vi "Actor Core.vi"(8 "error in":errorcluster, 11 "Dispatcher in":refnum<class "Dispatcher.lvclass">) -> (0 "error out":errorcluster, 3 "Actor out":refnum<class "Actor.lvclass">)   [LabVIEW 2013, in "Dispatcher.lvclass"]
doc: "(<B>Filename</B>: Actor Framework.lvlib:Actor.lvclass:Actor Core.vi)\n\nReceives messages to the actor, reacts to them, and initiates any error handling that may shut the actor down.\n\nDescendant classes may override this VI to append parallel tasks for the actor to complete while it handles messages. Overrides use the Call Parent Method node."
uses:
  Dispatcher.lvclass
  <vilib>/ActorFramework/Actor/Actor.lvclass
  Receiver/Receiver.lvclass
  <vilib>/ActorFramework/Actor/Actor.lvclass/Actor.ctl
  <vilib>/ActorFramework/Message Enqueuer/Message Enqueuer.lvclass/Message Enqueuer.ctl
  Dispatcher.lvclass/Dispatcher.ctl
  <vilib>/ActorFramework/Message Enqueuer/Init from Existing Queue.vi
  <vilib>/ActorFramework/Message Enqueuer/Enqueue.vi
  <vilib>/ActorFramework/Message Priority Queue/Priority Enqueue.vi
  <vilib>/ActorFramework/Message Enqueuer/Message Enqueuer.lvclass
  <vilib>/ActorFramework/Stop Msg/Stop Msg.lvclass
  Receiver Messages/Hide Front Panel Msg/Hide Front Panel Msg.lvclass
  Receiver Messages/Show Front Panel Msg/Show Front Panel Msg.lvclass
panel:
  in  "Show Receiver":bool
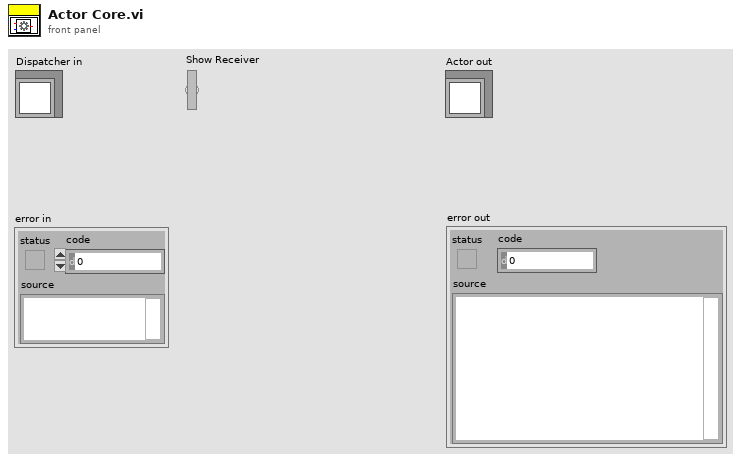
[diagram p1: front panel]
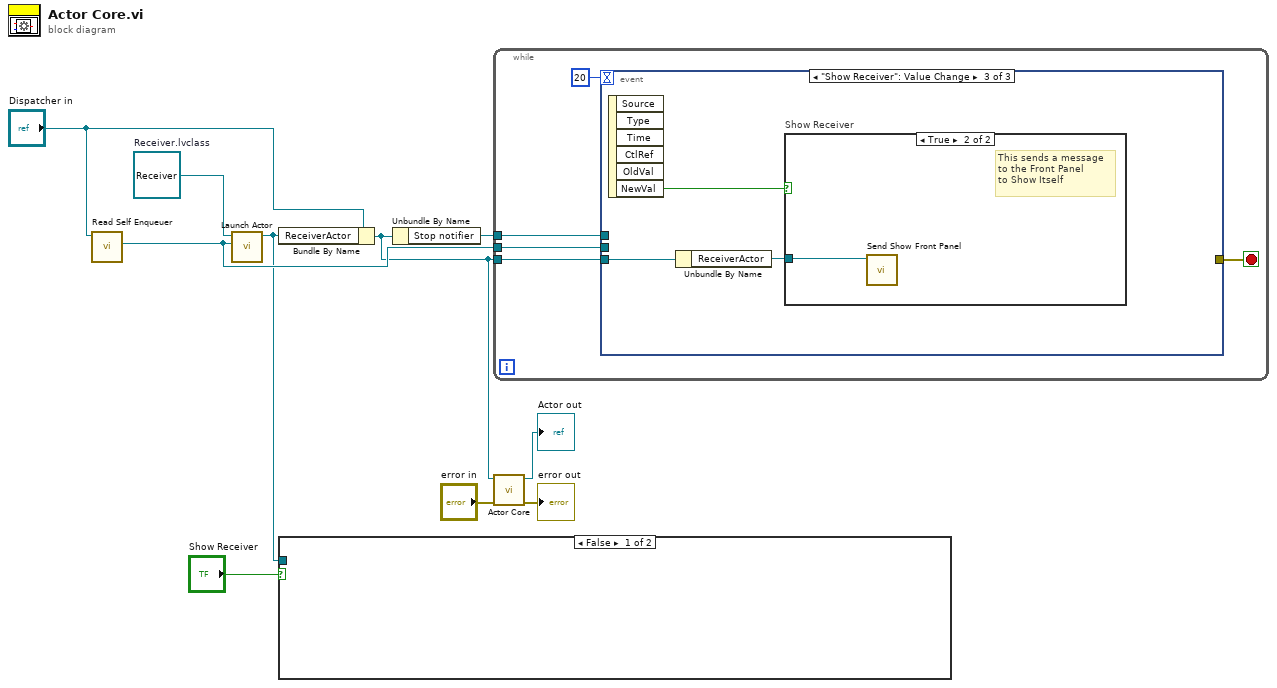
[diagram p0: block diagram]
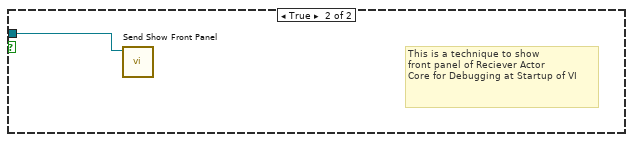
[diagram p2: hidden frame]
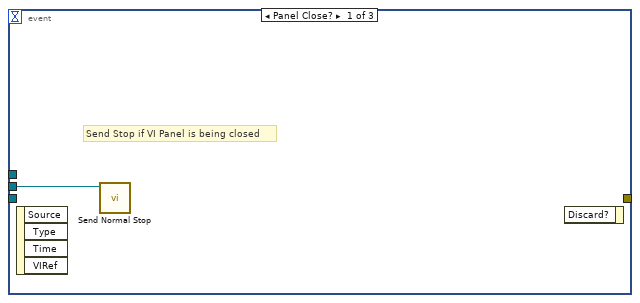
[diagram p3: hidden frame]
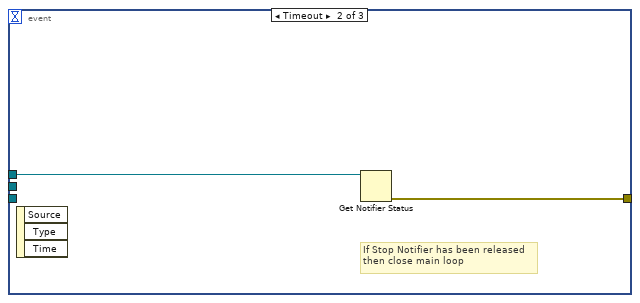
[diagram p4: hidden frame]
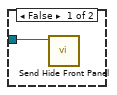
[diagram p5: hidden frame]
diagram:
  w4 = refnum<class "Receiver.lvclass"> refnum  # Receiver.lvclass
  n1 = call <vilib>:"Read Self Enqueuer.vi"("Actor"="Dispatcher in") -> ("Self Enqueuer"=w5:refnum<class "Message Enqueuer.lvclass">)  [unwired: 10 in]
  n2 = call <vilib>:"Launch Actor.vi"("Actor-to-Caller Enqueuer"=w5, "Actor"=w4) -> ("Caller-To-Actor Enqueuer"=w1:refnum<class "Message Enqueuer.lvclass">)  [unwired: 8 in, 1 out]
  n3 = Bundle By Name(cluster="Dispatcher in", "ReceiverActor"=w1) -> (w3:refnum<class "Dispatcher.lvclass">)
  n4 = case shown="False" "Show Receiver" {
    tunnel: w1 -> [_ w11]
    frame False {
    }
    frame True {
      # "This is a technique to show \nfront panel of Reciever Actor\nCore for Debugging at Startup of VI"
      n5 = call "Send Show Front Panel.vi"("Message Enqueuer"=w11) -> ()  [unwired: 9 in, 2 out]
    }
  }
  n6 = Unbundle By Name(w3) -> ("Stop notifier"=w7:refnum<notifier>)
  n7 = while {
    tunnel: w7 -> [w16]
    tunnel: w5 -> [w13]
    tunnel: w3 -> [w12]
    stop <- w15 stop-if-true
    n8 = event shown="[2] \"Show Receiver\": Value Change" {
      selector: _ -> [_ _ _]
      dyn-events: _ -> [_ _ _]
      timeout: 20 -> [_ _ _]
      tunnel: w16 -> [_ w19 _]
      tunnel: [_ w18 _] -> w15
      tunnel: w13 -> [w17 _ _]
      tunnel: w12 -> [_ _ w21]
      event Panel Close? {
        # "Send Stop if VI Panel is being closed"
        n9 = event-data() -> ()  [unwired: 1 in, 4 out]
        n10 = call <vilib>:"Send Normal Stop.vi"("Message Enqueuer"=w17) -> ()  [unwired: 10 in, 1 out]
        n11 = event-data() -> ()  [unwired: 2 in, 1 out]
      }
      event Timeout {
        # "If Stop Notifier has been released\nthen close main loop"
        n12 = event-data() -> ()  [unwired: 1 in, 3 out]
        n13 = Get Notifier Status(notifier=w19) -> (error out=w18:errorcluster)  [unwired: 1 in, 4 out]
      }
      event "Show Receiver": Value Change {
        n14 = event-data() -> ("NewVal"=w22:bool)  [unwired: 1 in, 5 out]
        n15 = Unbundle By Name(w21) -> ("ReceiverActor"=w20:refnum<class "Message Enqueuer.lvclass">)
        n16 = case "Show Receiver" shown="True" w22 {
          tunnel: w20 -> [w23 w24]
          frame False {
            n17 = call "Send Hide Front Panel.vi"("Message Enqueuer"=w23) -> ()  [unwired: 9 in, 2 out]
          }
          frame True {
            # "This sends a message \nto the Front Panel\nto Show Itself"
            n18 = call "Send Show Front Panel.vi"("Message Enqueuer"=w24) -> ()  [unwired: 9 in, 2 out]
          }
        }
      }
    }
  }
  n19 = call-parent "Actor Core.vi"("error in"="error in", "Actor in"=w3) -> ("error out"=→"error out":errorcluster, "Actor out"=→"Actor out":refnum<class "Actor.lvclass">)  [unwired: 8 in]
